vi "ResetDevice_SC.vi"(8 "error in (no error)":errorcluster, 11 "SysCfgDeployRequest":T1) -> (0 "error out":errorcluster)   [LabVIEW 2017]
uses:
  <vilib>/addons/InsightCM/MessageBus/MessageLibrary/SysCfgDeployer/controls/SysCfgDeployPackageRequestBody.ctl
  <vilib>/nisyscfg/Close (System).vi
  <vilib>/nisyscfg/nisyscfg.lvlib
panel:
  in  "Password":string
  in  "User Name":string="admin"
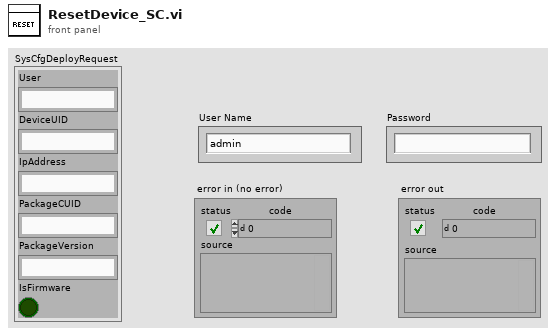
[diagram p1: front panel]
types:
  T1 = typedef "SysCfgDeployPackageRequestBody.ctl" = cluster{"User":string, "DeviceUID":string, "IpAddress":string, "PackageCUID":string, "PackageVersion":string, "IsFirmware":bool}
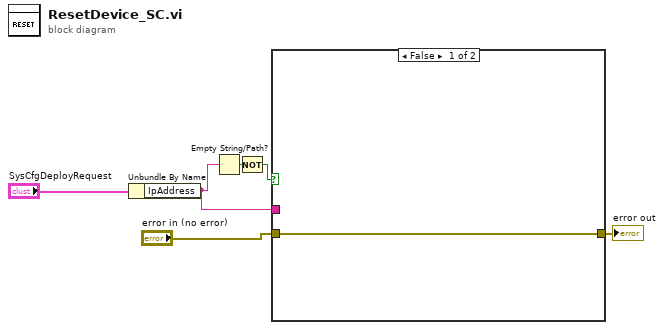
[diagram p0: block diagram]
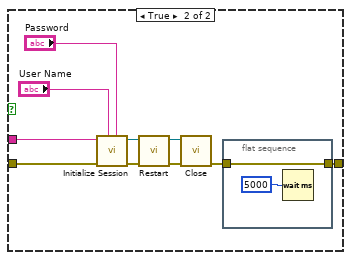
[diagram p2: hidden frame]
diagram:
  n1 = Unbundle By Name("SysCfgDeployRequest") -> ("IpAddress"=w1:string)
  n2 = Empty String/Path?(string/path=w1) -> (empty?=w2:bool)
  n3 = Not(x=w2) -> (.not. x?=w3:bool)
  n4 = case shown="False" w3 {
    tunnel: "error in (no error)" -> [w7 w17]
    tunnel: [w7 w10] -> w4
    tunnel: w1 -> [_ w8]
    frame False {
    }
    frame True {
      n5 = call <vilib>:"Initialize Session.vi"("Password"="Password", "User Name"="User Name", "error in (no error)"=w17, "Target (localhost)"=w8) -> ("error out"=w13:errorcluster, "Session out"=w12:refnum<k21>)  [unwired: 6 in]
      n6 = call <vilib>:"Restart.vi"("error in (no error)"=w13, "Session in"=w12) -> ("error out"=w11:errorcluster, "Session out"=w14:refnum<k21>)  [unwired: 7 in, 1 out]
      n7 = call-poly <vilib>:"Close.vi"("error in (no error)"=w11, "Session in"=w14) -> ("error out"=w9:errorcluster)  [unwired: 9 in]
      n8 = flat-sequence {
        tunnel: [w18] -> w10
        tunnel: w9 -> [w18]
        frame #0 {
          n9 = Wait (ms)(milliseconds to wait=u32 5000) -> ()  [unwired: 1 out]
        }
      }
    }
  }
  "error out" <- w4
